vi "Read Lines.vi"(8 "error in (no error)":errorcluster, 11 "SystemLin Tag Module configuration in":refnum<class "SystemLink File configuration.lvclass">) -> (0 "error out":errorcluster, 2 "Lines":T1[](array[typedef]), 3 "SystemLin Tag Module configuration out":refnum<class "SystemLink File configuration.lvclass">)   [LabVIEW 2015]
uses:
  SystemLink File configuration.lvclass
  <vilib>/NI/Tag Bus Module Framework/channel/TBM channel.lvclass
  Line.ctl
  Data Tag Type.ctl
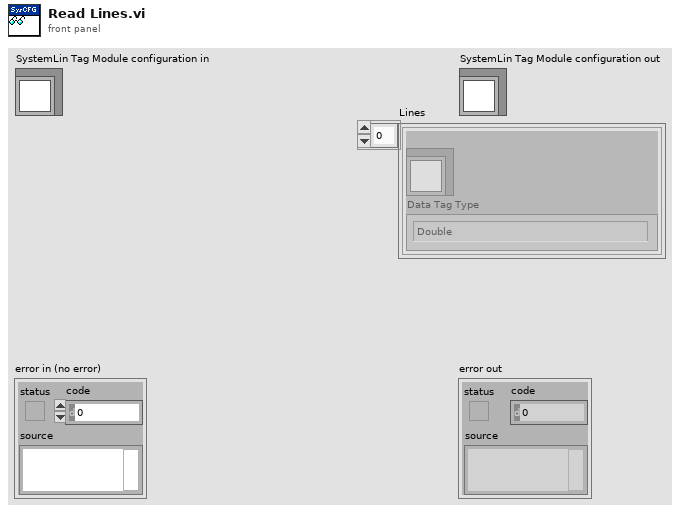
[diagram p1: front panel]
types:
  T1 = typedef "SystemLink File configuration.lvclass/Line.ctl" = cluster{"channel":refnum<class "TBM channel.lvclass">, "Data Tag Type":T2}
  T2 = typedef "SystemLink File configuration.lvclass/Data Tag Type.ctl" = enum16{"Double", "Single", "I32", "I16", "I8", "U64", "U32", "U16", "U8", "Boolean", "String", "Timestamp"}
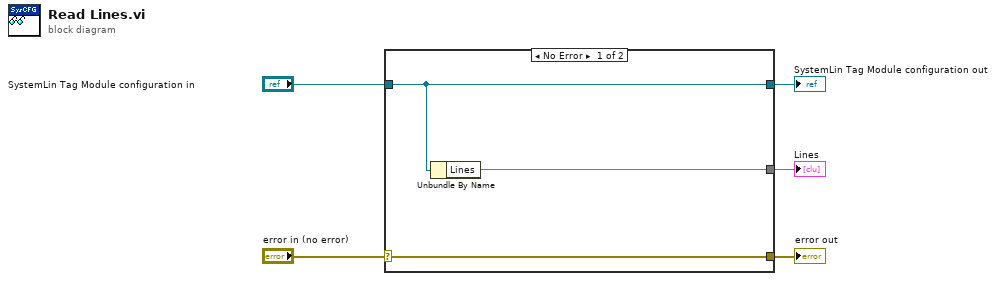
[diagram p0: block diagram]
diagram:
  n1 = case shown="No Error" "error in (no error)" {
    selector: "error in (no error)" -> [w8 w9]
    tunnel: [w8 w9] -> w4
    tunnel: [w7 w10] -> w2
    tunnel: "SystemLin Tag Module configuration in" -> [w7 w10]
    tunnel: [w6 _] -> w1
    frame No Error {
      n2 = Unbundle By Name(w7) -> ("Lines"=w6)
    }
    frame Error {
    }
  }
  "error out" <- w4
  "SystemLin Tag Module configuration out" <- w2
  "Lines" <- w1
